vi "oa_Unwrap Wrap Phase in XY Signal (N Channels).vi"(6 "view":T1={"dB on? (F)"=FALSE, "unwrap phase? (T)"=TRUE, "unit in degree? (T)"=TRUE}, 7 "reset? (F)":bool, 9 "Unwrap?":bool, 11 "XY signals":cluster{"X":dbl[], "Y":dbl[]}[](array[cluster]) {"X" format="%.2f"; "Y" format="%.2f"}) -> (3 "XY signals out":cluster{"X":dbl[], "Y":dbl[]}[](array[cluster]) {"X" format="%.2f"; "Y" format="%.2f"})   [LabVIEW 2017, in "SoundVib_OAUtility.lvlib"]
uses:
  <vilib>/addons/Sound and Vibration/Order Analysis/Utility/SoundVib_OAUtility.lvlib
  <vilib>/addons/Sound and Vibration/Order Analysis/Misc/OAT Convert Phase (1 channel).vi
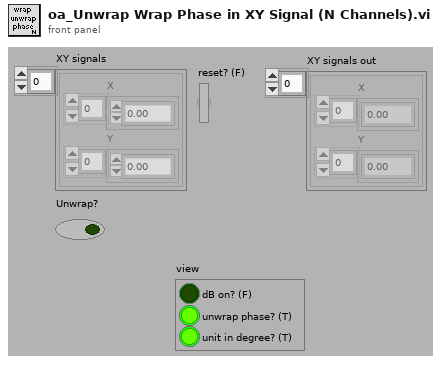
[diagram p1: front panel]
types:
  T1 = cluster{"dB on? (F)":bool, "unwrap phase? (T)":bool, "unit in degree? (T)":bool}
  T2 = cluster{"Unwrap?":bool, "unit in degree? (T)":bool}
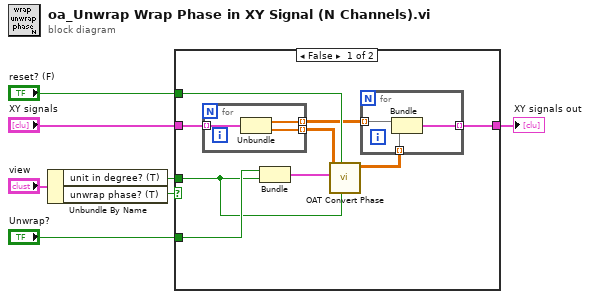
[diagram p0: block diagram]
diagram:
  n1 = Unbundle By Name("view") -> ("unit in degree? (T)"=w3:bool, "unwrap phase? (T)"=w6:bool)
  n2 = case shown="False" w6 {
    tunnel: "XY signals" -> [w16 w23]
    tunnel: [w15 w23] -> w4
    tunnel: w3 -> [w8 _]
    tunnel: "reset? (F)" -> [w14 _]
    tunnel: "Unwrap?" -> [w12 _]
    frame False {
      n3 = for {
        tunnel: w16 -> [w22] mode=indexing
        tunnel: [w21] -> w13 mode=indexing
        tunnel: [w20] -> w11 mode=indexing
        n4 = Unbundle(w22) -> ("X"=w21:dbl[], "Y"=w20:dbl[])
      }
      n5 = Bundle("Unwrap?"=w12, "unit in degree? (T)"=w8) -> (w9:T2)  [unwired: 1 in]
      n6 = call-poly <vilib>:"OAT Convert Phase.vi"("input unit in degree?"=w8, "reset (TRUE)"=w14, "desired phase setting"=w9, "phase in (rad)"=w11) -> ("phase out"=w10:dbl[][])  [unwired: 7 in]
      n7 = for {
        tunnel: [w19] -> w15 mode=indexing
        tunnel: w13 -> [w18] mode=indexing
        tunnel: w10 -> [w17] mode=indexing
        n8 = Bundle("X"=w18, "phase out"=w17) -> (w19:cluster{"X":dbl[], "phase out":dbl[]})  [unwired: 1 in]
      }
    }
    frame True {
    }
  }
  "XY signals out" <- w4
